vi "Autonomous Independent.vi"() -> ()   [LabVIEW 2012]
doc: "This VI is called when autonomous begins, and will automatically be terminated when autonomous ends. You can carry out timed or sensor driven robot movement independently without needing to return to the caller."
uses:
  <vilib>/Rock Robotics/WPI/Solenoid/WPI_SolenoidValue.ctl
  Robot Global Data.vi
  <vilib>/Rock Robotics/WPI/RobotDrive/WPI_RobotDriveGetSetRefNum.vi
  <vilib>/Rock Robotics/WPI/Solenoid/WPI_SolenoidSetEnum.vi
  <vilib>/Rock Robotics/WPI/Joystick/WPI_JoystickGetSetRefNum.vi
  <vilib>/Rock Robotics/WPI/RobotDrive/WPI_RobotDriveArcadeDrive_Standard(NoSaturation).vi
panel:
  out "Current Movement, for debugging":T1 {"Y Joystick Value" scale=1.0..-1.0; "X Joystick Value" scale=-1.0..1.0}
  in  "Array of robot movements":T2(array[cluster]) {"Y Joystick Value" scale=1.0..-1.0; "X Joystick Value" scale=-1.0..1.0}
  # "Be sure to right-click and choose Data Operations>>Make Current Value default if you want to save the array values with the VI"
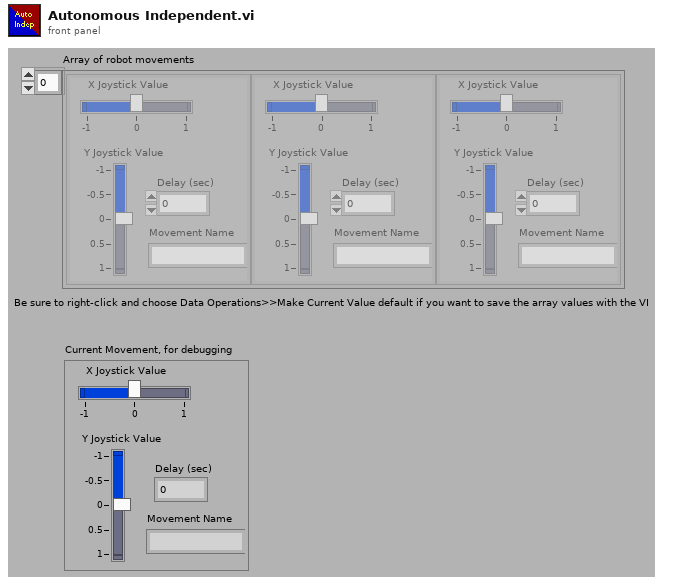
[diagram p1: front panel]
types:
  T1 = cluster{"X Joystick Value":dbl, "Y Joystick Value":dbl, "Delay (sec)":dbl, "Movement Name":string}
  T2 = cluster{"X Joystick Value":dbl, "Y Joystick Value":dbl, "Delay (sec)":dbl, "Movement Name":string}[]
  T3 = typedef "WPI_RobotDriveDevRef.ctl" = cluster{"DevStatus":errorcluster, "Motors[]":T4[], "Square Inputs":bool, "Max Output":dbl, "Isochronous":bool}
  T4 = typedef "WPI_MotorControlDeviceRef.ctl" = cluster{"DeviceStatus":errorcluster, "Type":enum16{"PWM", "CAN"}, "PWM":cluster{"Digital Module":T5, "PWM Channel":T6, "DeadBand":T7}, "CAN":cluster{"Device Number":u8, "Control Mode":T8, "Semaphore":T9, "Max Vout":dbl}, "Invert":bool, "TransformRef":T10, "InvTransformRef":T10}
  T5 = typedef "FPGA_TypedefDigitalModule.ctl" = enum16{"Digital Module 1", "Digital Module 2"}
  T6 = typedef "FPGA_DIOPWMChannel.ctl" = enum8{"PWM 1", "PWM 2", "PWM 3", "PWM 4", "PWM 5", "PWM 6", "PWM 7", "PWM 8", "PWM 9", "PWM 10", "Invalid"}
  T7 = typedef "WPI_PWMDeadband.ctl" = cluster{"Name":string, "maxPositivePwm":i32, "minPositivePwm":i32, "centerPwm":i32, "maxNegativePwm":i32, "minNegativePwm":i32, "angularRange":u16}
  T8 = typedef "WPI_CANJaguar_ControlMode.ctl" = enum8{"Percent VBus", "Current", "Speed", "Position", "Voltage"}
  T9 = typedef "Semaphore RefNum" = refnum<k1>
  T10 = typedef "WPI_PWMTransform_ConPane.ctl" = refnum<vi>
  T11 = typedef "WPI_JoystickDevRef.ctl" = cluster{"Device":T12}
  T12 = typedef "WPI_JoystickDeviceEnum.ctl" = enum16{"USB 1", "USB 2", "USB 3", "USB 4", "Kinect 1", "Kinect 2"}
  T13 = typedef "WPI_SolenoidValue.ctl" = enum16{"Off", "On", "Forward", "Reverse"}
  T14 = typedef "WPI_SolenoidDevRef.ctl" = cluster{"DevStatus":errorcluster, "Solenoid Module":T15, "Forward Solenoid Channel":T16, "Reverse Solenoid Channel":T16}
  T15 = typedef "FPGA_TypedefSolenoidModule.ctl" = enum16{"Solenoid Module 1", "Solenoid Module 2"}
  T16 = typedef "WPI_SolenoidChannel.ctl" = enum8{"Solenoid 1", "Solenoid 2", "Solenoid 3", "Solenoid 4", "Solenoid 5", "Solenoid 6", "Solenoid 7", "Solenoid 8", "Invalid"}
  T17 = cluster{"axis 1 (x)":dbl, "axis 2 (y)":dbl, "axis 3 (throttle)":dbl, "axis 4":dbl, "axis 5":dbl, "axis 6":dbl}
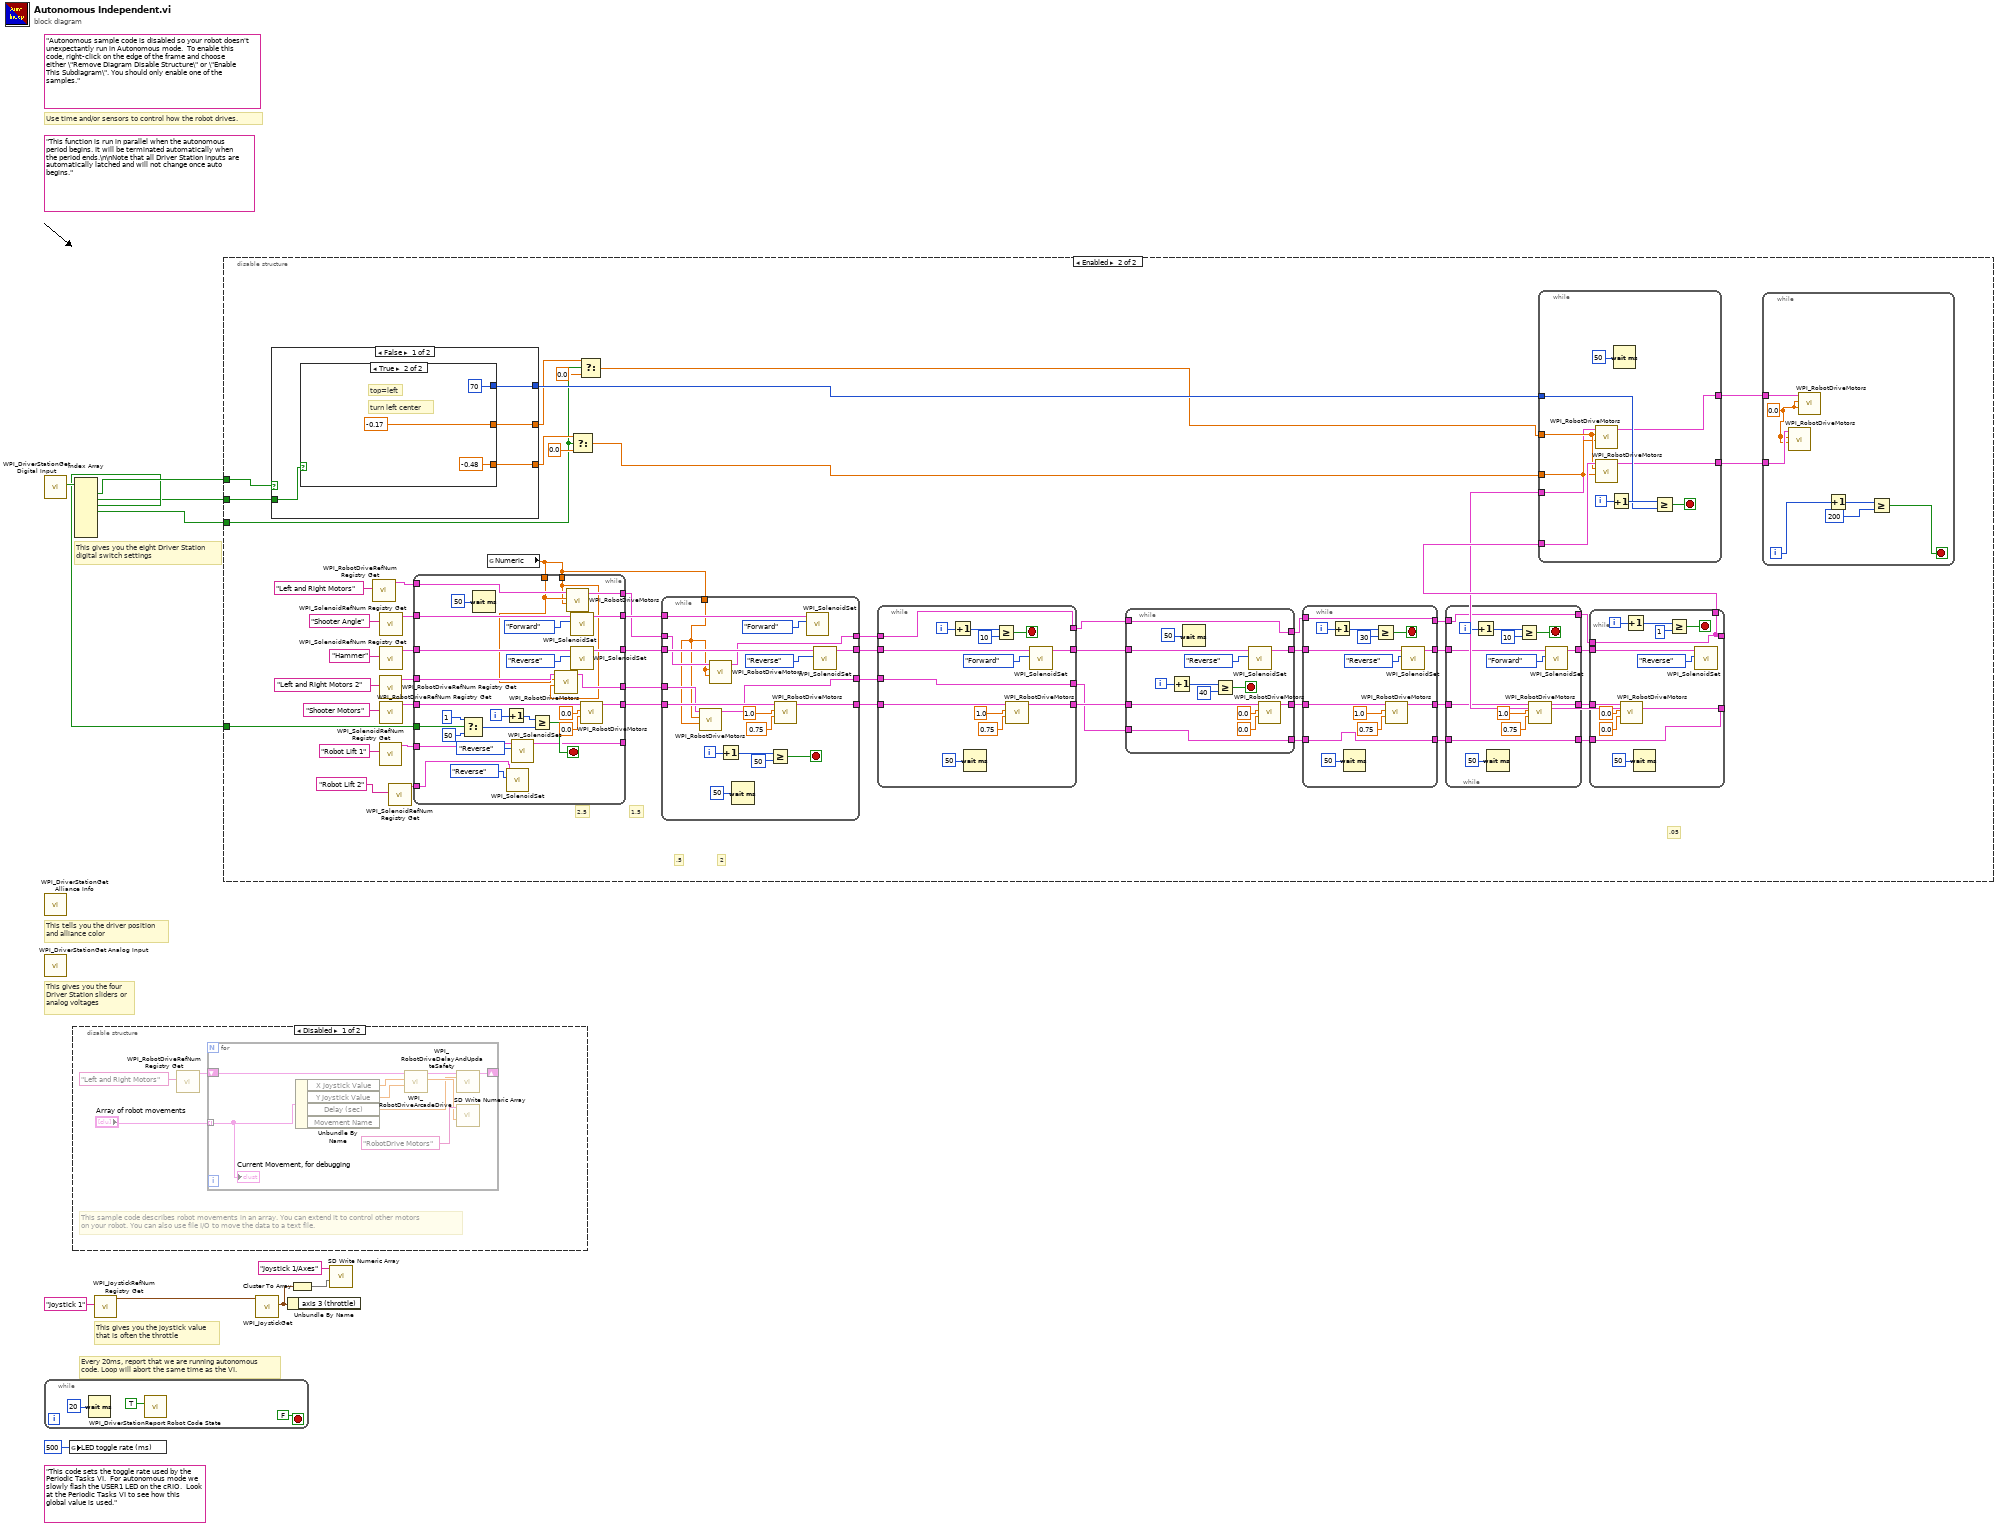
[diagram p0: block diagram]
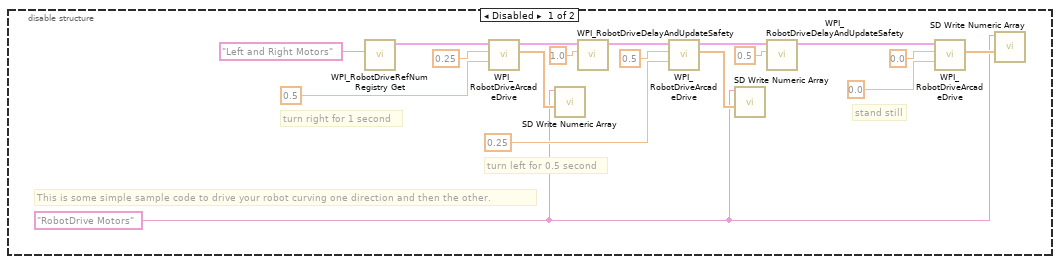
[diagram p3: hidden frame]
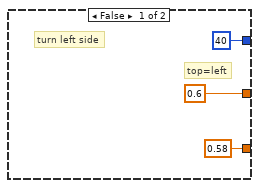
[diagram p4: hidden frame]
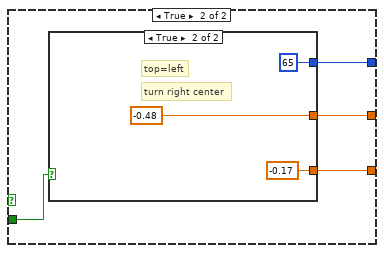
[diagram p5: hidden frame]
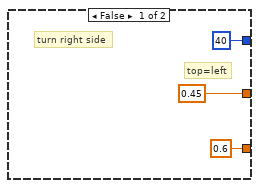
[diagram p6: hidden frame]
diagram:
  (unwired) "This code sets the toggle rate used by the Periodic Tasks VI.  For autonomous mode we slowly flash the USER1 LED on the cRIO.  Look at the Periodic Tasks VI to see how this global value is used."
  (unwired) "Autonomous sample code is disabled so your robot doesn't unexpectantly run in Autonomous mode.  To enable this code, right-click on the edge of the frame and choose either \"Remove Diagram Disable Structure\" or \"Enable This Subdiagram\". You should only enable one of the samples."
  (unwired) "This function is run in parallel when the autonomous period begins. It will be terminated automatically when the period ends.\n\nNote that all Driver Station inputs are automatically latched and will not change once auto begins."
  # "Every 20ms, report that we are running autonomous\ncode. Loop will abort the same time as the VI."
  # "This gives you the joystick value\nthat is often the throttle"
  # "Use time and/or sensors to control how the robot drives."
  # "This tells you the driver position\nand alliance color"
  # "This gives you the eight Driver Station\ndigital switch settings"
  # "This gives you the four\nDriver Station sliders or\nanalog voltages"
  n1 = call <vilib>:"WPI_DriverStationGet Digital Input.vi"() -> ("Driver Station Digital Input (1-8)"=w11:bool[])  [unwired: 11 out]
  n2 = call <vilib>:"WPI_DriverStationGet Alliance Info.vi"() -> ()  [unwired: 12 out]
  n3 = call <vilib>:"WPI_DriverStationGet Analog Input.vi"() -> ()  [unwired: 12 out]
  n4 = while {
    stop <- FALSE stop-if-true
    n5 = Wait (ms)(milliseconds to wait=u32 20) -> ()  [unwired: 1 out]
    n6 = call <vilib>:"WPI_DriverStationReport Robot Code State.vi"("Autonomous"=TRUE) -> ()  [unwired: 10 in, 1 out]
  }
  n7 = global write "Robot Global Data.vi" "LED toggle rate (ms)"(u32 500 ("LED ms toggle rate")) -> ()
  n8 = disable-structure shown="Disabled" {
    frame Disabled {
      # "This sample code describes robot movements in an array. You can extend it to control other motors\non your robot. You can also use file I/O to move the data to a text file."
      n9 = call <vilib>:"WPI_RobotDriveRefNum Registry Get.vi"("refnum name"="Left and Right Motors") -> ("RobotDriveDevRef"=w16:T3)  [unwired: 1 in, 9 out]
      n10 = for {
        shift-right: [w22] -> _
        shift-left: w16 -> [w23]
        tunnel: "Array of robot movements" -> [w18] mode=indexing
        n11 = Unbundle By Name(w18) -> ("X Joystick Value"=w21:dbl, "Y Joystick Value"=w20:dbl, "Delay (sec)"=w19:dbl)  [unwired: 1 out]
        n12 = call-poly <vilib>:"WPI_RobotDriveArcadeDrive.vi"("Y axis value"=w20, "X axis value"=w21, "RobotDriveDevRef"=w23) -> ("Motor Values"=w25:dbl[], "RobotDriveDevRef"=w24:T3)  [unwired: 1 in, 6 out]
        n13 = call <vilib>:"WPI_RobotDriveDelayAndUpdateSafety.vi"("Delay (s)"=w19, "RobotDriveDevRef"=w24) -> ("RobotDriveDevRef 2"=w22:T3)  [unwired: 8 in, 1 out]
        n14 = call <vilib>:"SD Write Numeric Array.vi"("Numeric Array"=w25, "Name"="RobotDrive Motors") -> ()  [unwired: 8 in, 2 out]
        "Current Movement, for debugging" <- w18
      }
    }
    frame Enabled {
    }
  }
  n15 = Index Array(array=w11) -> (element #1=w4:bool, element #2=w2:bool, element #3=w3:bool, element #4=w1:bool)  [unwired: 8 in, 4 out]
  n16 = call <vilib>:"WPI_JoystickRefNum Registry Get.vi"("refnum name"="Joystick 1") -> ("JoystickDevRef"=w9:T11)  [unwired: 1 in, 9 out]
  n17 = disable-structure shown="Enabled" {
    disable-tunnel: w3 -> [_ w79]
    disable-tunnel: w4 -> [_ w86]
    disable-tunnel: w2 -> [_ w78]
    disable-tunnel: w1 -> [_ w54]
    frame Disabled {
      w27 = "RobotDrive Motors" ("Name")
      # "This is some simple sample code to drive your robot curving one direction and then the other."
      # "stand still"
      # "turn left for 0.5 second"
      # "turn right for 1 second"
      n18 = call <vilib>:"WPI_RobotDriveRefNum Registry Get.vi"("refnum name"="Left and Right Motors") -> ("RobotDriveDevRef"=w31:T3)  [unwired: 1 in, 9 out]
      n19 = call-poly <vilib>:"WPI_RobotDriveArcadeDrive.vi"("Y axis value"=0.5 ("X axis value"), "X axis value"=0.25, "RobotDriveDevRef"=w31) -> ("Motor Values"=w30:dbl[], "RobotDriveDevRef"=w38:T3)  [unwired: 1 in, 6 out]
      n20 = call <vilib>:"SD Write Numeric Array.vi"("Numeric Array"=w30, "Name"=w27) -> ()  [unwired: 8 in, 2 out]
      n21 = call <vilib>:"WPI_RobotDriveDelayAndUpdateSafety.vi"("Delay (s)"=1.0, "RobotDriveDevRef"=w38) -> ("RobotDriveDevRef 2"=w37:T3)  [unwired: 8 in, 1 out]
      n22 = call-poly <vilib>:"WPI_RobotDriveArcadeDrive.vi"("Y axis value"=0.25 ("X axis value"), "X axis value"=0.5, "RobotDriveDevRef"=w37) -> ("Motor Values"=w29:dbl[], "RobotDriveDevRef"=w36:T3)  [unwired: 1 in, 6 out]
      n23 = call <vilib>:"SD Write Numeric Array.vi"("Numeric Array"=w29, "Name"=w27) -> ()  [unwired: 8 in, 2 out]
      n24 = call <vilib>:"WPI_RobotDriveDelayAndUpdateSafety.vi"("Delay (s)"=0.5, "RobotDriveDevRef"=w36) -> ("RobotDriveDevRef 2"=w35:T3)  [unwired: 8 in, 1 out]
      n25 = call-poly <vilib>:"WPI_RobotDriveArcadeDrive.vi"("Y axis value"=0.0 ("X axis value"), "X axis value"=0.0, "RobotDriveDevRef"=w35) -> ("Motor Values"=w28:dbl[])  [unwired: 1 in, 7 out]
      n26 = call <vilib>:"SD Write Numeric Array.vi"("Numeric Array"=w28, "Name"=w27) -> ()  [unwired: 8 in, 2 out]
    }
    frame Enabled {
      # ".05"
      # "1.5"
      # "2"
      # ".5"
      # "2.5"
      n27 = case shown="False" w86 {
        tunnel: w78 -> [w150 w160]
        tunnel: [w148 w159] -> w56
        tunnel: [w149 w158] -> w51
        tunnel: [w147 w157] -> w75
        frame False {
          n28 = case shown="True" w150 {
            tunnel: [0.6 ("X axis value") -0.17 ("X axis value")] -> w149
            tunnel: [0.58 ("RightSpeed") -0.48 ("RightSpeed")] -> w148
            tunnel: [40 70] -> w147
            frame False {
              # "turn left side"
              # "top=left"
            }
            frame True {
              # "top=left"
              # "turn left center"
            }
          }
        }
        frame True {
          n29 = case shown="True" w160 {
            tunnel: [0.45 ("X axis value") -0.48 ("X axis value")] -> w158
            tunnel: [0.6 ("RightSpeed") -0.17 ("RightSpeed")] -> w159
            tunnel: [40 65] -> w157
            frame False {
              # "turn right side"
              # "top=left"
            }
            frame True {
              # "top=left"
              # "turn right center"
            }
          }
        }
      }
      n30 = call <vilib>:"WPI_RobotDriveRefNum Registry Get.vi"("refnum name"="Left and Right Motors") -> ("RobotDriveDevRef"=w74:T3)  [unwired: 1 in, 9 out]
      n31 = call <vilib>:"WPI_RobotDriveRefNum Registry Get.vi"("refnum name"="Left and Right Motors 2") -> ("RobotDriveDevRef"=w64:T3)  [unwired: 1 in, 9 out]
      n32 = call <vilib>:"WPI_SolenoidRefNum Registry Get.vi"("refnum name"="Robot Lift 1") -> ("SolenoidDevRef"=w48:T14)  [unwired: 9 in, 1 out]
      n33 = call <vilib>:"WPI_SolenoidRefNum Registry Get.vi"("refnum name"="Shooter Angle") -> ("SolenoidDevRef"=w85:T14)  [unwired: 9 in, 1 out]
      n34 = call <vilib>:"WPI_SolenoidRefNum Registry Get.vi"("refnum name"="Hammer") -> ("SolenoidDevRef"=w82:T14)  [unwired: 9 in, 1 out]
      n35 = call <vilib>:"WPI_RobotDriveRefNum Registry Get.vi"("refnum name"="Shooter Motors") -> ("RobotDriveDevRef"=w81:T3)  [unwired: 1 in, 9 out]
      n36 = call <vilib>:"WPI_SolenoidRefNum Registry Get.vi"("refnum name"="Robot Lift 2") -> ("SolenoidDevRef"=w46:T14)  [unwired: 9 in, 1 out]
      n37 = global read "Robot Global Data.vi" "Numeric"() -> (w50:dbl)
      n38 = while {
        tunnel: [w136] -> w84
        tunnel: w85 -> [w137]
        tunnel: [w139] -> w83
        tunnel: w82 -> [w138]
        tunnel: w81 -> [w134]
        tunnel: [w135] -> w80
        tunnel: w79 -> [w130]
        tunnel: [w127] -> w73
        tunnel: w74 -> [w128]
        tunnel: [w125] -> w65
        tunnel: w64 -> [w126]
        tunnel: w50 -> [w124]
        tunnel: w50 -> [w123]
        tunnel: w48 -> [w122]
        tunnel: [w120] -> _
        tunnel: w46 -> [w118]
        i -> [w129]
        stop <- w140 stop-if-true
        n39 = Select(t=1, s=w130, f=50 ("y")) -> (s? t:f=w131:i32)
        n40 = Wait (ms)(milliseconds to wait=u32 50) -> ()  [unwired: 1 out]
        n41 = Increment(x=w129) -> (x+1=w144:i32)
        n42 = call-poly <vilib>:"WPI_SolenoidSet.vi"("Value"=WPI_SolenoidValue."Reverse", "SolenoidDevRef"=w118) -> ()  [unwired: 8 in, 2 out]
        n43 = call-poly <vilib>:"WPI_SolenoidSet.vi"("Value"=WPI_SolenoidValue."Reverse", "SolenoidDevRef"=w122) -> ("SolenoidDevRef"=w120:T14)  [unwired: 8 in, 1 out]
        n44 = Greater Or Equal?(x=w144, y=w131) -> (x >= y?=w140:bool)
        n45 = call <vilib>:"WPI_RobotDriveMotors.vi"("RightSpeed"=w123, "LeftSpeed"=w124, "RobotDriveDevRef"=w126) -> ("RobotDriveDevRef"=w125:T3)  [unwired: 6 in, 2 out]
        n46 = call <vilib>:"WPI_RobotDriveMotors.vi"("RightSpeed"=w123, "LeftSpeed"=w124, "RobotDriveDevRef"=w128) -> ("RobotDriveDevRef"=w127:T3)  [unwired: 6 in, 2 out]
        n47 = call-poly <vilib>:"WPI_SolenoidSet.vi"("Value"=WPI_SolenoidValue."Forward", "SolenoidDevRef"=w137) -> ("SolenoidDevRef"=w136:T14)  [unwired: 8 in, 1 out]
        n48 = call-poly <vilib>:"WPI_SolenoidSet.vi"("Value"=WPI_SolenoidValue."Reverse", "SolenoidDevRef"=w138) -> ("SolenoidDevRef"=w139:T14)  [unwired: 8 in, 1 out]
        n49 = call <vilib>:"WPI_RobotDriveMotors.vi"("RightSpeed"=0.0, "LeftSpeed"=0.0 ("X axis value"), "RobotDriveDevRef"=w134) -> ("RobotDriveDevRef"=w135:T3)  [unwired: 6 in, 2 out]
      }
      n50 = Select(t=w56, s=w54, f=0.0) -> (s? t:f=w45:dbl)
      n51 = Select(t=w51, s=w54, f=0.0) -> (s? t:f=w52:dbl)
      n52 = while {
        tunnel: w80 -> [w251]
        tunnel: w83 -> [w250]
        tunnel: [w245] -> w97
        tunnel: [w244] -> w96
        tunnel: w84 -> [w241]
        tunnel: w73 -> [w239]
        tunnel: [w238] -> w72
        tunnel: [w237] -> w66
        tunnel: w65 -> [w236]
        tunnel: w50 -> [w235]
        i -> [w246]
        stop <- w247 stop-if-true
        n53 = call <vilib>:"WPI_RobotDriveMotors.vi"("RightSpeed"=w235, "LeftSpeed"=w235, "RobotDriveDevRef"=w236) -> ("RobotDriveDevRef"=w237:T3)  [unwired: 6 in, 2 out]
        n54 = call <vilib>:"WPI_RobotDriveMotors.vi"("RightSpeed"=w235, "LeftSpeed"=w235, "RobotDriveDevRef"=w239) -> ("RobotDriveDevRef"=w238:T3)  [unwired: 6 in, 2 out]
        n55 = Increment(x=w246) -> (x+1=w248:i32)
        n56 = Wait (ms)(milliseconds to wait=u32 50) -> ()  [unwired: 1 out]
        n57 = Greater Or Equal?(x=w248, y=50) -> (x >= y?=w247:bool)
        n58 = call <vilib>:"WPI_RobotDriveMotors.vi"("RightSpeed"=0.75, "LeftSpeed"=1.0 ("X axis value"), "RobotDriveDevRef"=w251) -> ("RobotDriveDevRef"=w245:T3)  [unwired: 6 in, 2 out]
        n59 = call-poly <vilib>:"WPI_SolenoidSet.vi"("Value"=WPI_SolenoidValue."Forward", "SolenoidDevRef"=w241) -> ()  [unwired: 8 in, 2 out]
        n60 = call-poly <vilib>:"WPI_SolenoidSet.vi"("Value"=WPI_SolenoidValue."Reverse", "SolenoidDevRef"=w250) -> ("SolenoidDevRef"=w244:T14)  [unwired: 8 in, 1 out]
      }
      n61 = while {
        tunnel: w97 -> [w234]
        tunnel: w96 -> [w233]
        tunnel: [w226] -> w95
        tunnel: [w225] -> w94
        tunnel: [w222] -> w71
        tunnel: w72 -> [w222]
        tunnel: [w221] -> w60
        tunnel: w66 -> [w221]
        i -> [w228]
        stop <- w229 stop-if-true
        n62 = Increment(x=w228) -> (x+1=w232:i32)
        n63 = Wait (ms)(milliseconds to wait=u32 50) -> ()  [unwired: 1 out]
        n64 = Greater Or Equal?(x=w232, y=10) -> (x >= y?=w229:bool)
        n65 = call <vilib>:"WPI_RobotDriveMotors.vi"("RightSpeed"=0.75, "LeftSpeed"=1.0, "RobotDriveDevRef"=w234) -> ("RobotDriveDevRef"=w226:T3)  [unwired: 6 in, 2 out]
        n66 = call-poly <vilib>:"WPI_SolenoidSet.vi"("Value"=WPI_SolenoidValue."Forward", "SolenoidDevRef"=w233) -> ("SolenoidDevRef"=w225:T14)  [unwired: 8 in, 1 out]
      }
      n67 = while {
        tunnel: w95 -> [w220]
        tunnel: w94 -> [w219]
        tunnel: [w211] -> w93
        tunnel: [w210] -> w92
        tunnel: [w208] -> w70
        tunnel: w71 -> [w208]
        tunnel: [w207] -> w61
        tunnel: w60 -> [w207]
        i -> [w213]
        stop <- w214 stop-if-true
        n68 = Increment(x=w213) -> (x+1=w217:i32)
        n69 = Wait (ms)(milliseconds to wait=u32 50) -> ()  [unwired: 1 out]
        n70 = Greater Or Equal?(x=w217, y=40) -> (x >= y?=w214:bool)
        n71 = call-poly <vilib>:"WPI_SolenoidSet.vi"("Value"=WPI_SolenoidValue."Reverse", "SolenoidDevRef"=w219) -> ("SolenoidDevRef"=w210:T14)  [unwired: 8 in, 1 out]
        n72 = call <vilib>:"WPI_RobotDriveMotors.vi"("RightSpeed"=0.0, "LeftSpeed"=0.0, "RobotDriveDevRef"=w220) -> ("RobotDriveDevRef"=w211:T3)  [unwired: 6 in, 2 out]
      }
      n73 = while {
        tunnel: w93 -> [w206]
        tunnel: w92 -> [w205]
        tunnel: [w197] -> w91
        tunnel: [w196] -> w90
        tunnel: [w194] -> w69
        tunnel: w70 -> [w194]
        tunnel: [w193] -> w62
        tunnel: w61 -> [w193]
        i -> [w199]
        stop <- w200 stop-if-true
        n74 = Increment(x=w199) -> (x+1=w203:i32)
        n75 = Wait (ms)(milliseconds to wait=u32 50) -> ()  [unwired: 1 out]
        n76 = Greater Or Equal?(x=w203, y=30) -> (x >= y?=w200:bool)
        n77 = call <vilib>:"WPI_RobotDriveMotors.vi"("RightSpeed"=0.75, "LeftSpeed"=1.0, "RobotDriveDevRef"=w206) -> ("RobotDriveDevRef"=w196:T3)  [unwired: 6 in, 2 out]
        n78 = call-poly <vilib>:"WPI_SolenoidSet.vi"("Value"=WPI_SolenoidValue."Reverse", "SolenoidDevRef"=w205) -> ("SolenoidDevRef"=w197:T14)  [unwired: 8 in, 1 out]
      }
      n79 = while {
        tunnel: w90 -> [w192]
        tunnel: w91 -> [w191]
        tunnel: [w183] -> w89
        tunnel: [w182] -> w88
        tunnel: [w180] -> w68
        tunnel: w69 -> [w180]
        tunnel: [w179] -> w63
        tunnel: w62 -> [w179]
        i -> [w185]
        stop <- w186 stop-if-true
        n80 = Increment(x=w185) -> (x+1=w189:i32)
        n81 = Wait (ms)(milliseconds to wait=u32 50) -> ()  [unwired: 1 out]
        n82 = Greater Or Equal?(x=w189, y=10) -> (x >= y?=w186:bool)
        n83 = call <vilib>:"WPI_RobotDriveMotors.vi"("RightSpeed"=0.75, "LeftSpeed"=1.0, "RobotDriveDevRef"=w192) -> ("RobotDriveDevRef"=w183:T3)  [unwired: 6 in, 2 out]
        n84 = call-poly <vilib>:"WPI_SolenoidSet.vi"("Value"=WPI_SolenoidValue."Forward", "SolenoidDevRef"=w191) -> ("SolenoidDevRef"=w182:T14)  [unwired: 8 in, 1 out]
      }
      n85 = while {
        tunnel: w89 -> [w178]
        tunnel: w88 -> [w177]
        tunnel: [w168] -> _
        tunnel: w68 -> [w168]
        tunnel: [w168] -> w67
        tunnel: [w167] -> w59
        tunnel: w63 -> [w167]
        i -> [w171]
        stop <- w172 stop-if-true
        n86 = call <vilib>:"WPI_RobotDriveMotors.vi"("RightSpeed"=0.0, "LeftSpeed"=0.0, "RobotDriveDevRef"=w178) -> ()  [unwired: 6 in, 3 out]
        n87 = Increment(x=w171) -> (x+1=w175:i32)
        n88 = Wait (ms)(milliseconds to wait=u32 50) -> ()  [unwired: 1 out]
        n89 = Greater Or Equal?(x=w175, y=1) -> (x >= y?=w172:bool)
        n90 = call-poly <vilib>:"WPI_SolenoidSet.vi"("Value"=WPI_SolenoidValue."Reverse", "SolenoidDevRef"=w177) -> ()  [unwired: 8 in, 2 out]
      }
      n91 = while {
        tunnel: w67 -> [w114]
        tunnel: w52 -> [w113]
        tunnel: w45 -> [w112]
        tunnel: w75 -> [w111]
        tunnel: w59 -> [w110]
        tunnel: [w108] -> w58
        tunnel: [w107] -> w57
        i -> [w116]
        stop <- w115 stop-if-true
        n92 = call <vilib>:"WPI_RobotDriveMotors.vi"("RightSpeed"=w112, "LeftSpeed"=w113, "RobotDriveDevRef"=w110) -> ("RobotDriveDevRef"=w108:T3)  [unwired: 6 in, 2 out]
        n93 = call <vilib>:"WPI_RobotDriveMotors.vi"("RightSpeed"=w112, "LeftSpeed"=w113, "RobotDriveDevRef"=w114) -> ("RobotDriveDevRef"=w107:T3)  [unwired: 6 in, 2 out]
        n94 = Increment(x=w116) -> (x+1=w117:i32)
        n95 = Wait (ms)(milliseconds to wait=u32 50) -> ()  [unwired: 1 out]
        n96 = Greater Or Equal?(x=w117, y=w111) -> (x >= y?=w115:bool)
      }
      n97 = while {
        tunnel: w58 -> [w102]
        tunnel: w57 -> [w101]
        i -> [w104]
        stop <- w105 stop-if-true
        w100 = 0.0
        n98 = call <vilib>:"WPI_RobotDriveMotors.vi"("RightSpeed"=w100, "LeftSpeed"=w100, "RobotDriveDevRef"=w101) -> ()  [unwired: 6 in, 3 out]
        n99 = call <vilib>:"WPI_RobotDriveMotors.vi"("RightSpeed"=w100, "LeftSpeed"=w100, "RobotDriveDevRef"=w102) -> ()  [unwired: 6 in, 3 out]
        n100 = Increment(x=w104) -> (x+1=w106:i32)
        n101 = Greater Or Equal?(x=w106, y=200) -> (x >= y?=w105:bool)
      }
    }
  }
  n102 = call <vilib>:"WPI_JoystickGet.vi"("JoystickDevRef"=w9) -> ("Axes"=w6:T17)  [unwired: 1 in, 5 out]
  n103 = Unbundle By Name(w6) -> ()  [unwired: 1 out]
  n104 = Cluster To Array(cluster=w6) -> (array=w7:dbl[])
  n105 = call <vilib>:"SD Write Numeric Array.vi"("Numeric Array"=w7, "Name"="Joystick 1/Axes") -> ()  [unwired: 8 in, 2 out]
